vi "Setup subWorker - Oscilloscope.vi"(8 "error in":errorcluster, 11 "TopUI in":refnum<class "TopUI.lvclass">) -> (0 "error out":errorcluster, 3 "TopUI out":refnum<class "TopUI.lvclass">)   [LabVIEW 2025, in "TopUI.lvclass"]
doc: "This VI sets up the framework parameters of a statically-linked subWorker."
uses:
  TopUI.lvclass
  TopUI.lvclass/TopUI.ctl
  Oscilloscope/Oscilloscope.lvclass
  C:/Program Files (x86)/National Instruments/LabVIEW 2025/vi.lib/addons/_Workers/Library/Classes/Worker/Worker.lvclass
  C:/Program Files (x86)/National Instruments/LabVIEW 2025/vi.lib/addons/_Workers/Library/Classes/Workers Object/Workers Object.lvclass
  C:/Users/chrismadlax/Desktop/LVSampleCode/WorkersPolymorphism/Workers/Oscilloscope/Oscilloscope.lvclass
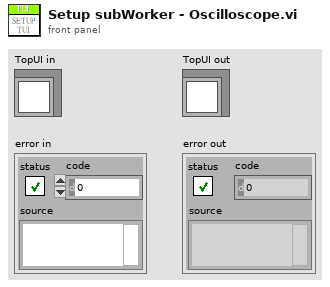
[diagram p1: front panel]
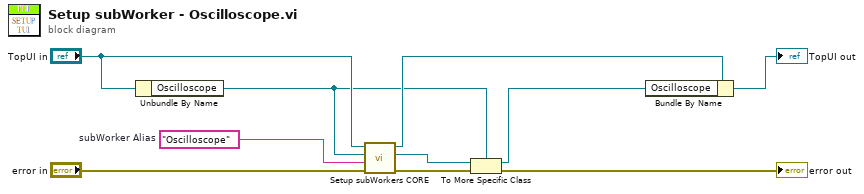
[diagram p0: block diagram]
diagram:
  w6 = "Oscilloscope"  # subWorker Alias
  n1 = Unbundle By Name("TopUI in") -> ("Oscilloscope"=w3:refnum<class "Oscilloscope.lvclass">)
  n2 = call-dynamic "Setup subWorkers CORE.vi"("error in"="error in", "subWorker Alias"=w6, "subWorker"=w3, "Worker"="TopUI in") -> ("error out"=w5:errorcluster, "subWorker out"=w1:refnum<class "Worker.lvclass">, "Worker out"=w8:refnum<class "TopUI.lvclass">)  [unwired: 5 in]
  n3 = To More Specific Class(target class=w3, reference=w1, error in=w5) -> (specific class reference=w2:refnum<class "Oscilloscope.lvclass">, error out=→"error out":errorcluster)
  n4 = Bundle By Name(cluster=w8, "Oscilloscope"=w2) -> (→"TopUI out":refnum<class "TopUI.lvclass">)
